vi "Write Module Error Configurations.vi"(7 "Module ID":string, 8 "error in":errorcluster, 10 "error responses":T1, 11 "Standard Engine Repo Data in":refnum<class "Standard Engine Configuration.lvclass">) -> (0 "error out":errorcluster, 3 "Standard Engine Repo Data out":refnum<class "Standard Engine Configuration.lvclass">)   [LabVIEW 2013, in "Standard Engine Configuration.lvclass"]
doc: "Specifies the error configuration for a specific module."
uses:
  Standard Engine Configuration.lvclass
  Runtime/error responses.ctl
  error options.ctl
  Standard Engine Configuration.lvclass/Standard Engine Configuration.ctl
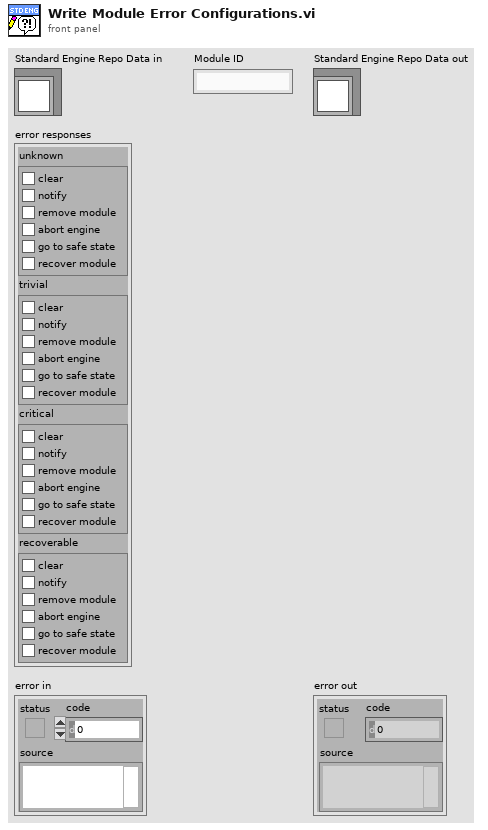
[diagram p1: front panel]
types:
  T1 = typedef "Standard Engine Configuration.lvclass/error responses.ctl" = cluster{"unknown":T2, "trivial":T2, "critical":T2, "recoverable":T2}
  T2 = typedef "Standard Engine Configuration.lvclass/error options.ctl" = cluster{"clear":bool, "notify":bool, "remove module":bool, "abort engine":bool, "go to safe state":bool, "recover module":bool}
  T3 = typedef "Standard Engine Configuration.lvclass/Module Specific Configuration.ctl" = cluster{"Module ID":string, "Module Decimation":T4, "error tag":string, "error responses":T1}
  T4 = typedef "Standard Engine Configuration.lvclass/Module Decimation.ctl" = cluster{"Decimation":u16, "Offset":u16, "sort order":i32, "async?":bool}
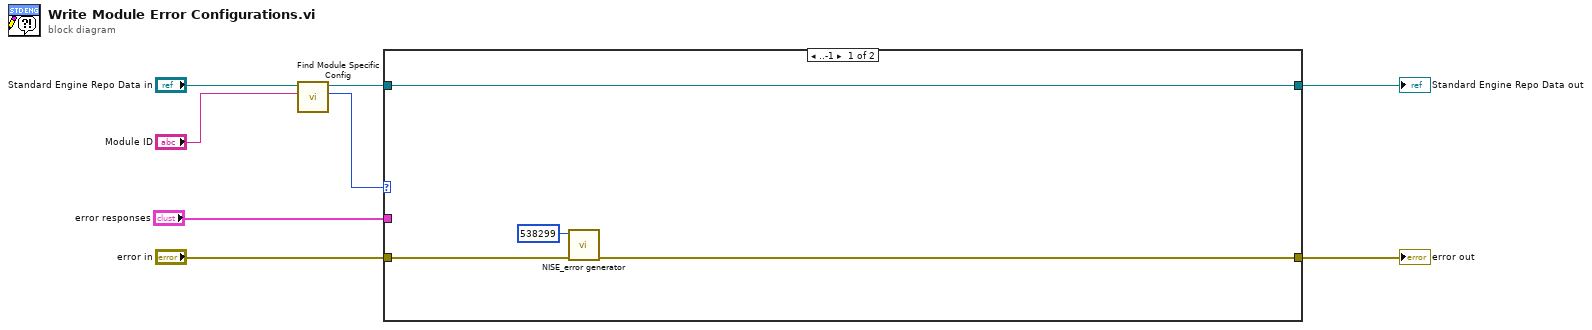
[diagram p0: block diagram]
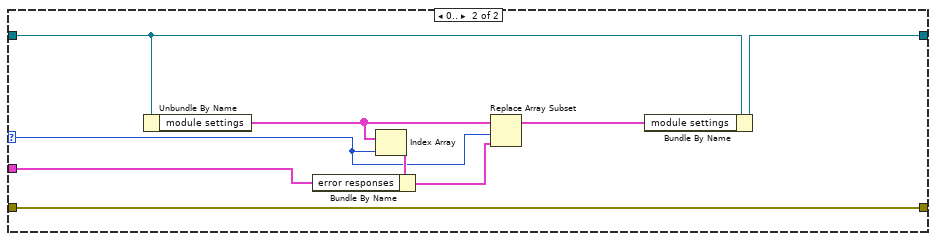
[diagram p2: hidden frame]
diagram:
  n1 = call "Find Module Specific Config.vi"("Module ID"="Module ID", "Standard Engine Repo Data in"="Standard Engine Repo Data in") -> ("Index"=w1:i32, "Standard Engine Repo Data out"=w2:refnum<class "Standard Engine Configuration.lvclass">)  [unwired: 8 in]
  n2 = case shown="..-1" w1 {
    selector: w1 -> [_ w19]
    tunnel: w2 -> [w11 w16]
    tunnel: "error in" -> [w12 w21]
    tunnel: [w10 w21] -> w4
    tunnel: [w11 w14] -> w5
    tunnel: "error responses" -> [_ w13]
    frame ..-1 {
      n3 = call <vilib>:"NISE_error generator.vi"("error in"=w12, "error code (0)"=538299) -> ("error out"=w10:errorcluster)  [unwired: 7 in]
    }
    frame 0.. {
      n4 = Unbundle By Name(w16) -> ("module settings"=w18:T3[])
      n5 = Index Array(array=w18, index=w19) -> (element=w20:T3)
      n6 = Bundle By Name(cluster=w20, "error responses"=w13) -> (w17:T3)
      n7 = Replace Array Subset(array=w18, new element=w17, index=w19) -> (w15:T3[])
      n8 = Bundle By Name(cluster=w16, "module settings"=w15) -> (w14:refnum<class "Standard Engine Configuration.lvclass">)
    }
  }
  "error out" <- w4
  "Standard Engine Repo Data out" <- w5
